vi "Write RefClkSource.vi"(8 "error in (no error)":errorcluster, 10 "RefClkSource":string="PXI_Trig0", 11 "PXI_MultiTrig in":refnum<class "PXI_MultiTrig.lvclass">) -> (0 "error out":errorcluster, 3 "PXI_MultiTrig out":refnum<class "PXI_MultiTrig.lvclass">)   [LabVIEW 2018, in "SyncPlugins.lvlib" / "PXI_MultiTrig.lvclass"]
uses:
  PXI_MultiTrig.lvclass
  PXI_MultiTrig.lvclass/PXI_MultiTrig.ctl
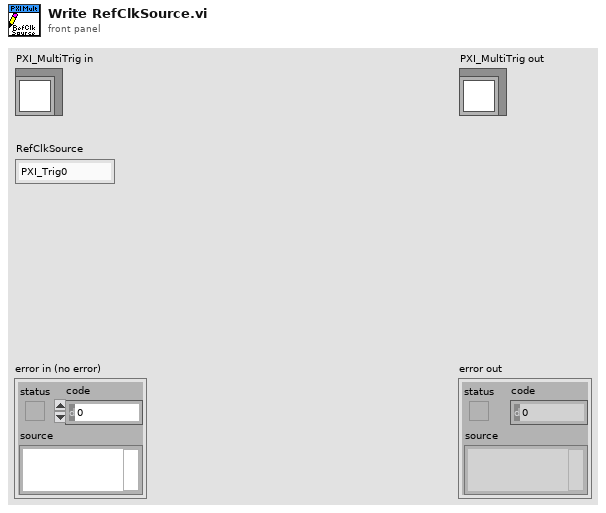
[diagram p1: front panel]
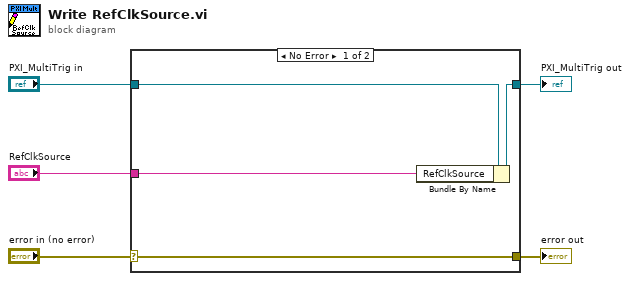
[diagram p0: block diagram]
diagram:
  n1 = case shown="No Error" "error in (no error)" {
    selector: "error in (no error)" -> [w9 w10]
    tunnel: [w9 w10] -> w4
    tunnel: [w7 w11] -> w2
    tunnel: "PXI_MultiTrig in" -> [w8 w11]
    tunnel: "RefClkSource" -> [w6 _]
    frame No Error {
      n2 = Bundle By Name(cluster=w8, "RefClkSource"=w6) -> (w7:refnum<class "PXI_MultiTrig.lvclass">)
    }
    frame Error {
    }
  }
  "error out" <- w4
  "PXI_MultiTrig out" <- w2
